vi "Edge Detector.vi"(0 "In":bool) -> (1 "Rising Edge":bool, 2 "Falling Edge":bool)   [LabVIEW 2025]
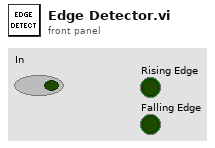
[diagram p1: front panel]
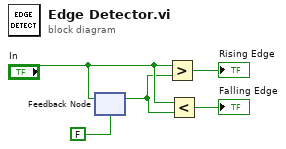
[diagram p0: block diagram]
diagram:
  n1 = feedback-in #1("In") -> ()
  n2 = feedback #1(FALSE ("In")) -> (w2:bool)
  n3 = Greater?(x="In", y=w2) -> (0:→"Rising Edge":bool)
  n4 = Less?(x="In", y=w2) -> (x < y?=→"Falling Edge":bool)
